vi "New Frame.vi"(8 "error in (no error)":errorcluster, 9 "Total Frames":i32, 10 "Current Frame":i32, 11 "Viewer in":refnum<class "Viewer.lvclass">) -> (0 "error out":errorcluster, 3 "Viewer out":refnum<class "Viewer.lvclass">)   [LabVIEW 2023, in "Viewer.lvlib" / "Viewer.lvclass"]
uses:
  Viewer.lvclass
  Viewer.lvclass/Viewer.ctl
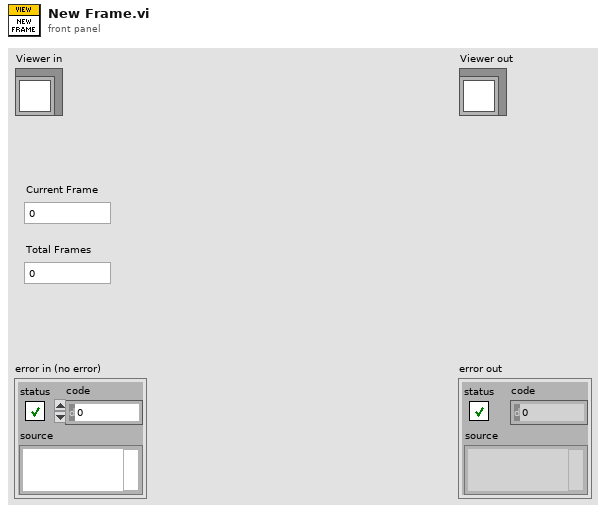
[diagram p1: front panel]
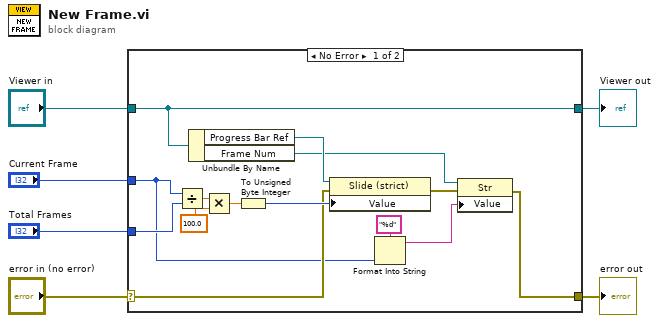
[diagram p0: block diagram]
diagram:
  n1 = case shown="No Error" "error in (no error)" {
    selector: "error in (no error)" -> [w13 w22]
    tunnel: [w7 w22] -> w5
    tunnel: [w20 w21] -> w3
    tunnel: "Viewer in" -> [w20 w21]
    tunnel: "Current Frame" -> [w9 _]
    tunnel: "Total Frames" -> [w14 _]
    frame No Error {
      n2 = Divide(x=w9, y=w14) -> (x/y=w18:dbl)
      n3 = Unbundle By Name(w20) -> ("Progress Bar Ref"=w19:refnum<vi>, "Frame Num"=w11:refnum<vi>)
      n4 = Multiply(x=w18, y=100.0) -> (x*y=w16:dbl)
      n5 = To Unsigned Byte Integer(number=w16) -> (unsigned 8bit integer=w15:u8)
      n6 = property class="Slide (strict)"(reference=w19, error in=w13, "Value"=w15) -> (error out=w12:errorcluster)  [unwired: 1 out]
      n7 = Format Into String(format string="%d", w9) -> (resulting string=w10:string)  [unwired: 2 in, 1 out]
      n8 = property class="Str"(reference=w11, error in=w12, "Value"=w10) -> (error out=w7:errorcluster)  [unwired: 1 out]
    }
    frame Error {
    }
  }
  "error out" <- w5
  "Viewer out" <- w3
